vi "Tests.vi"   [LabVIEW 2024, in "Tester InterComm.lvlib"]
uses:
  Tester InterComm.lvlib
  Queues - Destroy.vi
  References - Create.vi
  Queues - Create.vi
  References - Get.vi
  Queues - Get.vi
  References - Destroy.vi
  Tester Events - Create.vi
  Tester Events - Get.vi
  Tester Events - Register.vi
  Tester Events - Destroy.vi
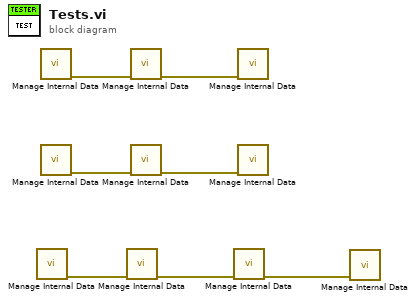
[diagram p0: block diagram]
diagram:
  n1 = call-poly "Manage Internal Data.vi"() -> ("error out"=w3:errorcluster)  [unwired: 11 in]
  n2 = call-poly "Manage Internal Data.vi"() -> ("error out"=w7:errorcluster)  [unwired: 11 in]
  n3 = call-poly "Manage Internal Data.vi"() -> ("error out"=w4:errorcluster)  [unwired: 11 in]
  n4 = call-poly "Manage Internal Data.vi"("error in"=w3) -> ("error out"=w2:errorcluster)  [unwired: 9 in, 1 out]
  n5 = call-poly "Manage Internal Data.vi"("error in"=w7) -> ("error out"=w6:errorcluster)  [unwired: 9 in, 1 out]
  n6 = call-poly "Manage Internal Data.vi"("error in"=w4) -> ("error out"=w5:errorcluster)  [unwired: 9 in, 1 out]
  n7 = call-poly "Manage Internal Data.vi"("error in"=w2) -> ("error out"=w1:errorcluster)  [unwired: 9 in, 1 out]
  n8 = call-poly "Manage Internal Data.vi"("error in"=w6) -> ()  [unwired: 10 in, 1 out]
  n9 = call-poly "Manage Internal Data.vi"("error in"=w5) -> ()  [unwired: 10 in, 1 out]
  n10 = call-poly "Manage Internal Data.vi"("error in"=w1) -> ()  [unwired: 10 in, 1 out]
